vi "SLASH.vi"(1 "3*3陣列":string[][](array[string])) -> (0 "O┪X墓":bool)   [LabVIEW 2014]
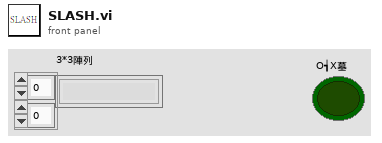
[diagram p1: front panel]
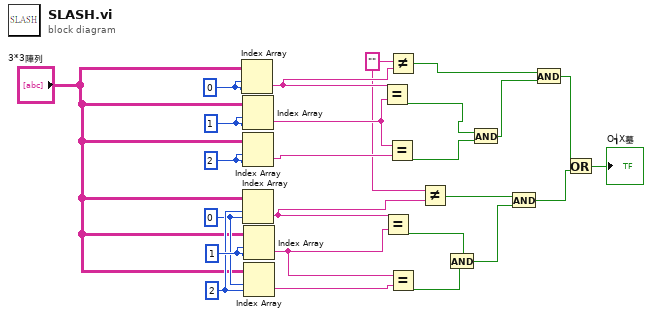
[diagram p0: block diagram]
diagram:
  w13 = 2
  w14 = 1
  w12 = 0
  w1 = ""
  w23 = 2
  w24 = 1
  w25 = 0
  n1 = Index Array(array="3*3陣列", index (row)=w25, index (col)=w25) -> (element=w18:string)
  n2 = Index Array(array="3*3陣列", index (row)=w24, index (col)=w24) -> (element=w22:string)
  n3 = Index Array(array="3*3陣列", index (row)=w23, index (col)=w23) -> (element=w5:string)
  n4 = Index Array(array="3*3陣列", index (row)=w13, index (col)=w12) -> (element=w6:string)
  n5 = Index Array(array="3*3陣列", index (row)=w14, index (col)=w14) -> (element=w8:string)
  n6 = Index Array(array="3*3陣列", index (row)=w12, index (col)=w13) -> (element=w7:string)
  n7 = Equal?(x=w18, y=w22) -> (x = y?=w21:bool)
  n8 = Equal?(x=w6, y=w8) -> (x = y?=w15:bool)
  n9 = Equal?(x=w22, y=w5) -> (x = y?=w20:bool)
  n10 = Not Equal?(x=w1, y=w18) -> (x != y?=w19:bool)
  n11 = Equal?(x=w8, y=w7) -> (x = y?=w16:bool)
  n12 = Not Equal?(x=w1, y=w6) -> (x != y?=w17:bool)
  n13 = And(x=w15, y=w16) -> (x .and. y?=w11:bool)
  n14 = And(x=w21, y=w20) -> (x .and. y?=w2:bool)
  n15 = And(x=w17, y=w11) -> (x .and. y?=w3:bool)
  n16 = And(x=w19, y=w2) -> (x .and. y?=w4:bool)
  n17 = Or(x=w4, y=w3) -> (x .or. y?=→"O┪X墓":bool)
